vi "WriteDataCsv.vi"(0 "session in":refnum<k35>, 7 "Array Results":string[](array[string]), 11 "error in":errorcluster) -> (4 "session out":refnum<k35>, 15 "error out":errorcluster)   [LabVIEW 2021]
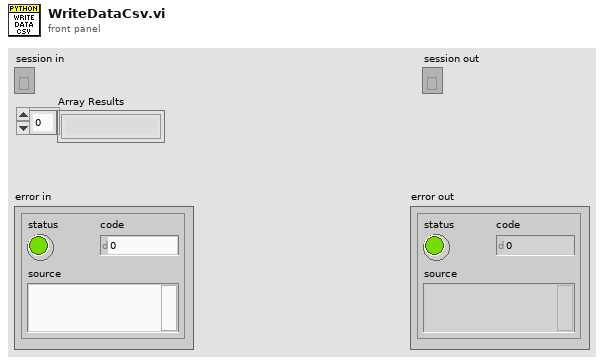
[diagram p1: front panel]
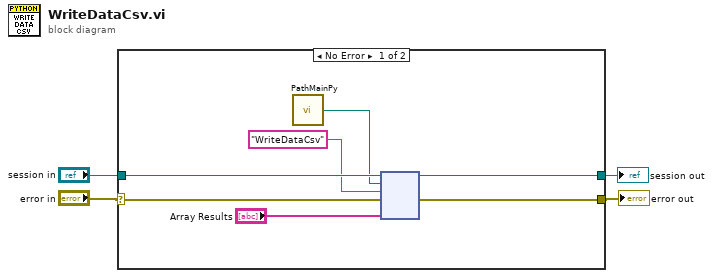
[diagram p0: block diagram]
diagram:
  n1 = case shown="No Error" "error in" {
    selector: "error in" -> [w11 w13]
    tunnel: [w9 w13] -> w1
    tunnel: "session in" -> [w10 w12]
    tunnel: [w8 w12] -> w3
    frame No Error {
      n2 = call "PathMainPy.vi"() -> ("path"=w6:path)  [unwired: 15 in]
      n3 = node(w10, w6, "WriteDataCsv" ("function name"), w11, "Array Results") -> (w8:refnum<k35>, w9:errorcluster)  [unwired: 3 in, 2 out]
    }
    frame Error {
    }
  }
  "session out" <- w3
  "error out" <- w1
